vi "Read Password.vi"(8 "error in (no error)":errorcluster, 11 "Master in":refnum<class "MASTER.lvclass">) -> (0 "error out":errorcluster, 3 "Master out":refnum<class "MASTER.lvclass">)   [LabVIEW 2014, in "Files Library.lvlib" / "Master.lvclass"]
uses:
  MASTER/MASTER.lvclass
  MASTER/MASTER.lvclass/MASTER.ctl
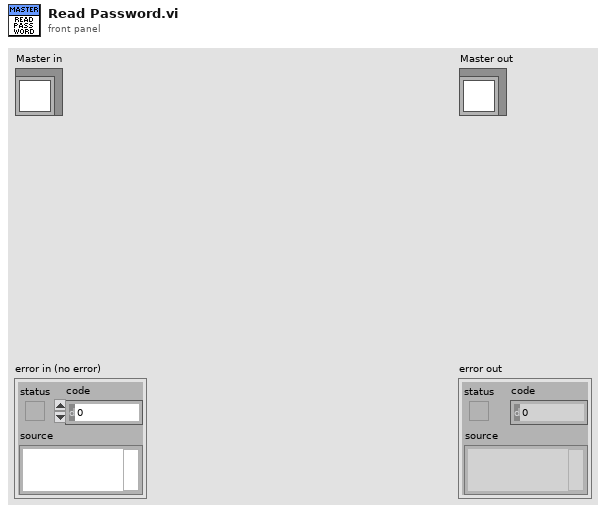
[diagram p1: front panel]
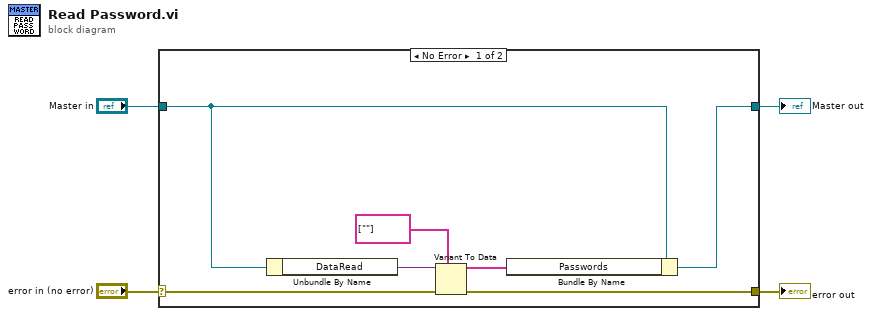
[diagram p0: block diagram]
diagram:
  n1 = case shown="No Error" "error in (no error)" {
    selector: "error in (no error)" -> [w10 w13]
    tunnel: [w9 w13] -> w3
    tunnel: [w6 w12] -> w1
    tunnel: "Master in" -> [w8 w12]
    frame No Error {
      n2 = Unbundle By Name(w8) -> ("DataRead"=w11:variant)
      n3 = Variant To Data(error in=w10, type=string[] [""], Variant=w11) -> (data=w7:string[], error out=w9:errorcluster)
      n4 = Bundle By Name(cluster=w8, "Passwords"=w7) -> (w6:refnum<class "MASTER.lvclass">)
    }
    frame Error {
    }
  }
  "error out" <- w3
  "Master out" <- w1
